vi "Sensor_Layout.vi"(8 "error in":errorcluster, 11 "camera handle in":u64) -> (0 "error out":errorcluster, 1 "Sensor_Layout":T1, 3 "camera handle out":u64)   [LabVIEW 2014, in "PICam.lvlib"]
doc: "ActiveWidth Controls the active number of columns.\nActiveHeight Controls the active number of rows.\nActiveLeftMargin Controls the inactive number of columns on the left.\nActiveTopMargin Controls the inactive number of rows on the top.\nActiveRightMargin Controls the inactive number of columns on the right.\nActiveBottomMargin Controls the inactive number of rows on the bottom."
uses:
  PICam.lvlib
  Ctrls/Sensor_Layout.ctl
  Program Files/Princeton Instruments/PICam/Runtime/Picam32.dll
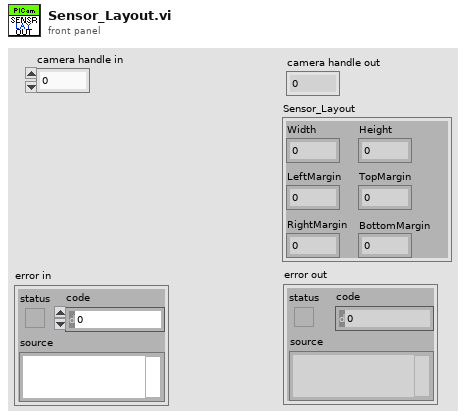
[diagram p1: front panel]
types:
  T1 = typedef "PICam.lvlib/Sensor_Layout.ctl" = cluster{"Width":i32, "Height":i32, "LeftMargin":i32, "TopMargin":i32, "RightMargin":i32, "BottomMargin":i32}
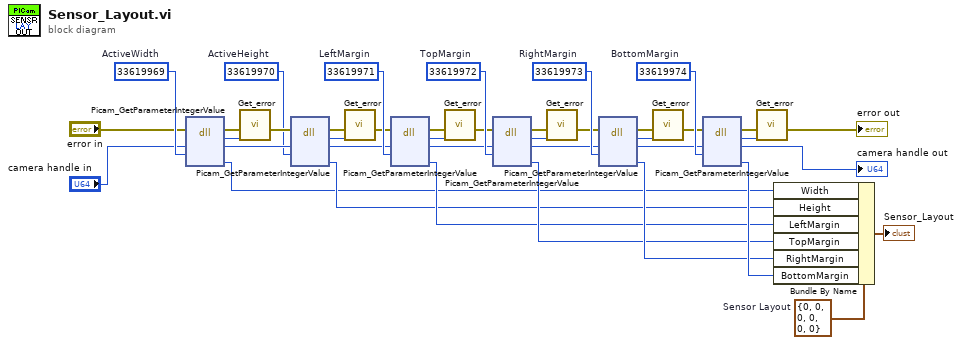
[diagram p0: block diagram]
diagram:
  w8 = T1 {"Width"=0, "Height"=0, "LeftMargin"=0, "TopMargin"=0, "RightMargin"=0, "BottomMargin"=0}  # Sensor Layout
  w16 = u32 33619974  # BottomMargin
  w22 = u32 33619973  # RightMargin
  w24 = u32 33619972  # TopMargin
  w30 = u32 33619971  # LeftMargin
  w31 = u32 33619970  # ActiveHeight
  w38 = u32 33619969  # ActiveWidth
  n1 = dll-call lib="C:/Program Files/Princeton Instruments/PICam/Runtime/Picam32.dll" fn="Picam_GetParameterIntegerValue"(error in="error in", "camera"="camera handle in", "PicamParameter"=w38) -> (error out=w40:errorcluster, "return type"=w39:i32, "camera"=w32:u64, "ActiveWidth"=w2:i32)  [unwired: 4 in, 1 out]
  n2 = call "Get_error.vi"("PICam_Error"=w39, "error in (no error)"=w40) -> ("error out"=w33:errorcluster)  [unwired: 9 in]
  n3 = dll-call lib="C:/Program Files/Princeton Instruments/PICam/Runtime/Picam32.dll" fn="Picam_GetParameterIntegerValue"(error in=w33, "camera"=w32, "PicamParameter"=w31) -> (error out=w34:errorcluster, "return type"=w35:i32, "camera"=w14:u64, "ActiveHeight"=w3:i32)  [unwired: 4 in, 1 out]
  n4 = call "Get_error.vi"("PICam_Error"=w35, "error in (no error)"=w34) -> ("error out"=w27:errorcluster)  [unwired: 9 in]
  n5 = dll-call lib="C:/Program Files/Princeton Instruments/PICam/Runtime/Picam32.dll" fn="Picam_GetParameterIntegerValue"(error in=w27, "camera"=w14, "PicamParameter"=w30) -> (error out=w29:errorcluster, "return type"=w28:i32, "camera"=w13:u64, "LeftMargin"=w4:i32)  [unwired: 4 in, 1 out]
  n6 = call "Get_error.vi"("PICam_Error"=w28, "error in (no error)"=w29) -> ("error out"=w23:errorcluster)  [unwired: 9 in]
  n7 = dll-call lib="C:/Program Files/Princeton Instruments/PICam/Runtime/Picam32.dll" fn="Picam_GetParameterIntegerValue"(error in=w23, "camera"=w13, "PicamParameter"=w24) -> (error out=w25:errorcluster, "return type"=w26:i32, "camera"=w12:u64, "TopMargin"=w5:i32)  [unwired: 4 in, 1 out]
  n8 = call "Get_error.vi"("PICam_Error"=w26, "error in (no error)"=w25) -> ("error out"=w19:errorcluster)  [unwired: 9 in]
  n9 = dll-call lib="C:/Program Files/Princeton Instruments/PICam/Runtime/Picam32.dll" fn="Picam_GetParameterIntegerValue"(error in=w19, "camera"=w12, "PicamParameter"=w22) -> (error out=w21:errorcluster, "return type"=w20:i32, "camera"=w11:u64, "RightMargin"=w6:i32)  [unwired: 4 in, 1 out]
  n10 = call "Get_error.vi"("PICam_Error"=w20, "error in (no error)"=w21) -> ("error out"=w15:errorcluster)  [unwired: 9 in]
  n11 = dll-call lib="C:/Program Files/Princeton Instruments/PICam/Runtime/Picam32.dll" fn="Picam_GetParameterIntegerValue"(error in=w15, "camera"=w11, "PicamParameter"=w16) -> (error out=w17:errorcluster, "return type"=w18:i32, "camera"=→"camera handle out":u64, "BottomMargin"=w7:i32)  [unwired: 4 in, 1 out]
  n12 = call "Get_error.vi"("PICam_Error"=w18, "error in (no error)"=w17) -> ("error out"=→"error out":errorcluster)  [unwired: 9 in]
  n13 = Bundle By Name(cluster=w8, "Width"=w2, "Height"=w3, "LeftMargin"=w4, "TopMargin"=w5, "RightMargin"=w6, "BottomMargin"=w7) -> (→"Sensor_Layout":T1)
